vi "panel2.vi"(8 "error in (no error)":errorcluster) -> (0 "error out":errorcluster)   [LabVIEW 2017]
uses:
  c24bc6ec-3696-4cc9-95ec-dee3b3b0cf5c.vi
  a288a1d7-2791-4915-a0b1-330fddf74d70.vi
  0919d1f0-e5d2-482b-8841-45466cc748b4.vi
  TagDB/_Support/DataAccess/_NameCacher.vi
  TagDB/_Support/Error/_[error50002]Invalid DataType.vi
  TagDB/_Support/Error/_[error50000]Invalid DB REF.vi
  TagDB/_Support/DataAccess/TagDB Ref to DVR.vi
  TagDB/_Support/URL/TRIM-BOTH-SPACE.vi
  TagDB/_Support/Error/_Build Error Cluster.vi
  TagDB/TagDB.lvlib
panel:
  out "value 2":variant
  out "Test send message":string
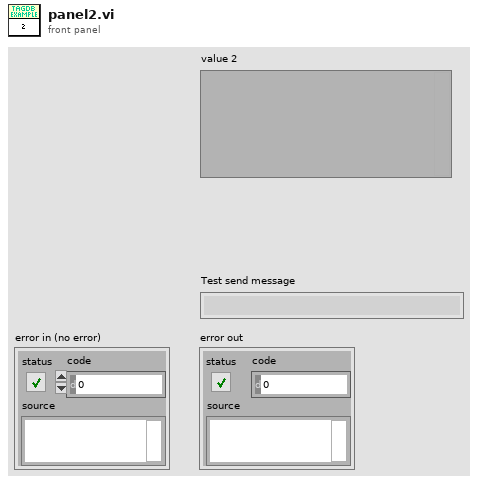
[diagram p1: front panel]
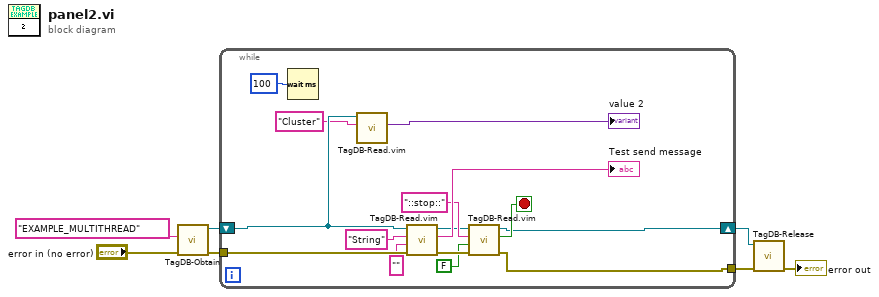
[diagram p0: block diagram]
diagram:
  n1 = call "TagDB-Obtain.vi"("error in (no error)"="error in (no error)", "name (unnamed)"="EXAMPLE_MULTITHREAD") -> ("error out"=w5:errorcluster, "TagDB"=w4:refnum<k1>)  [unwired: 3 in, 1 out]
  n2 = while {
    tunnel: w5 -> [w20]
    tunnel: [w13] -> w6
    shift-right: [w14] -> w1
    shift-left: w4 -> [w12]
    stop <- w18 stop-if-true
    n3 = Wait (ms)(milliseconds to wait=u32 100) -> ()  [unwired: 1 out]
    n4 = call "TagDB-Read.vim"("name"="Cluster", "TagDB"=w12) -> ("Value"=→"value 2":variant)  [unwired: 4 in, 5 out]
    n5 = call "TagDB-Read.vim"("error in (no error)"=w20, "Type(empty to read as variant)"="", "name"="String", "TagDB"=w12) -> ("error out"=w15:errorcluster, "Value"=→"Test send message":string, "TagDB(dup)"=w16:refnum<k1>)  [unwired: 2 in, 3 out]
    n6 = call "TagDB-Read.vim"("error in (no error)"=w15, "Type(empty to read as variant)"=FALSE, "name"="::stop::", "TagDB"=w16) -> ("error out"=w13:errorcluster, "Value"=w18:bool, "TagDB(dup)"=w14:refnum<k1>)  [unwired: 2 in, 3 out]
  }
  n7 = call "TagDB-Release.vi"("error in (no error)"=w6, "TagDB"=w1) -> ("error out"=→"error out":errorcluster)  [unwired: 9 in]
